vi "set_parameter_debug.vi"(6 "timeout (25000ms)":i32=25000, 8 "error in (no error)":errorcluster, 10 "Array":string[](array[string]), 11 "daemon reference in":refnum<k5>) -> (0 "error out":errorcluster, 2 "response":string, 3 "daemon reference out":refnum<k5>, 5 "command out":string="random")   [LabVIEW 2017]
doc: "<b>Command: </b>\"set_parameter\"\n\n<b>Description: </b> Instructs the target to set the specified parameter values.\n\n<b>Parameters: </b> \n\n 1. Parameter Array [max 20]\n 2. Value Array\n____________________________________________\nDIPC 692 Daemon API 10.0.0.1\nSam Tee - Dyson Technology Ltd\nCopyright (c) 2024, Dyson Technology Ltd"
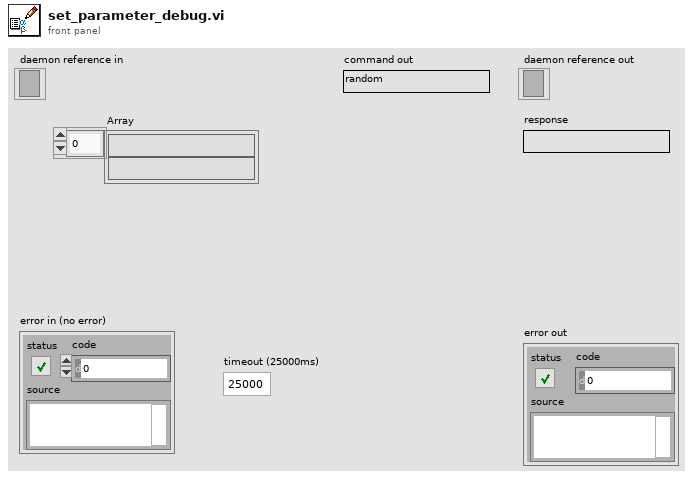
[diagram p1: front panel]
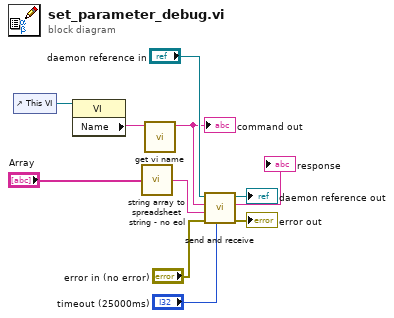
[diagram p0: block diagram]
diagram:
  n1 = control-ref of="This VI"() -> (w6:refnum<vi>)
  n2 = property class="VI"(reference=w6) -> ("Name"=w5:string)  [unwired: 1 in, 2 out]
  n3 = call "string array to spreadsheet string - no eol.vi"("string array"="Array") -> ("spreadsheet string - no eol"=w3:string)
  n4 = call "get vi name.vi"("library.lvlib:name.vi"=w5) -> ("vi name"=w4:string)  [unwired: 10 in]
  "command out" <- w4
  n5 = call "send and receive.vi"("timeout (25000ms)"="timeout (25000ms)", "error in (no error)"="error in (no error)", "data"=w3, "command"=w4, "daemon reference in"="daemon reference in") -> ("error out"=→"error out":errorcluster, "response"=→"response":string, "daemon reference out"=→"daemon reference out":refnum<k5>)  [unwired: 4 in]
